vi "Get Collision Type.vi"(7 "Combination in":string[](array[string]), 9 "GB Components in":refnum<class "Game Board Component.lvclass">[](array[class]), 11 "Game Board Component in":refnum<class "Game Board Component.lvclass">) -> (2 "Collision out":refnum<class "Collision.lvclass">, 5 "Combination out":string[](array[string]))   [LabVIEW 2024, in "Game Board Component.lvclass"]
doc: "MIT Licence\nCopyright (c) 2024 David Grollier"
uses:
  Game Board Component.lvclass
  Collision/Collision.lvclass
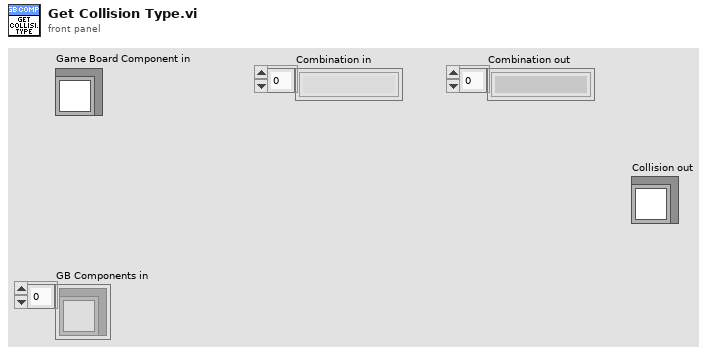
[diagram p1: front panel]
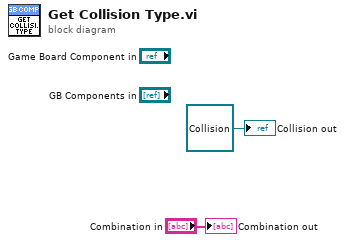
[diagram p0: block diagram]
diagram:
  "Collision out" <- refnum<class "Collision.lvclass"> refnum ("s? t:f")
  "Combination out" <- "Combination in"
